vi "Initialize.vi"(8 "error in (no error)":errorcluster, 10 "Reply to":refnum<class "Result Reply Msg.lvclass">, 11 "Measure Controller in":refnum<class "Process Controller.lvclass">) -> (0 "error out":errorcluster, 3 "Measure Controller out":refnum<class "Process Controller.lvclass">)   [LabVIEW 2016, in "Process Controller.lvclass"]
uses:
  Process Controller.lvclass
  Measure Object Messages/Result Reply Msg/Result Reply Msg.lvclass
  Process Controller Messages/Init Response Msg/Init Response Msg.lvclass
  D:/github/Measure_core/Measure Object Messages/Result Reply Msg/Result Reply Msg.lvclass
  Results/Acquired Result/Acquired Result.lvclass
  Measure Object Messages/Initialize Msg/Initialize Msg.lvclass/Initialize Msg.ctl
  <vilib>/ActorFramework/Message Enqueuer/Message Enqueuer.lvclass/Message Enqueuer.ctl
  Process Controller.lvclass/Process Controller.ctl
  <vilib>/ActorFramework/Message Enqueuer/Enqueue.vi
  Measure Object Messages/Initialize Msg/Initialize Msg.lvclass
  D:/Program Files/National Instruments/LabVIEW 2016/vi.lib/ActorFramework/Message/Message.lvclass
  <vilib>/ActorFramework/Message Priority Queue/Priority Enqueue.vi
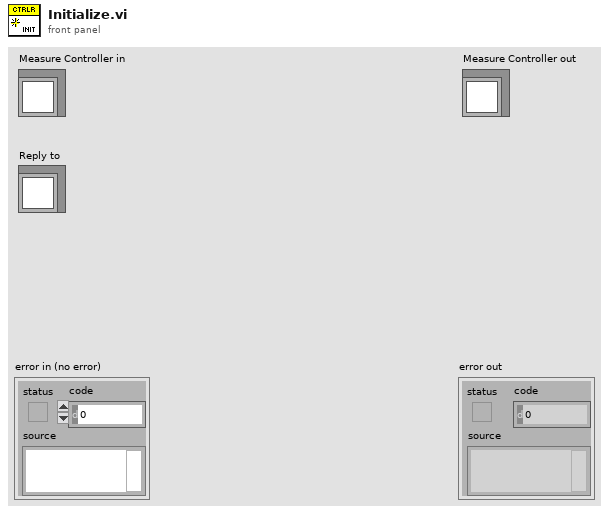
[diagram p1: front panel]
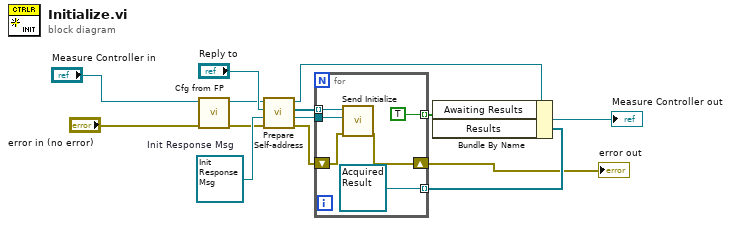
[diagram p0: block diagram]
diagram:
  w5 = refnum<class "Init Response Msg.lvclass"> refnum  # Init Response Msg
  n1 = call-dynamic "Cfg from FP.vi"("error in (no error)"="error in (no error)", "Measure Object in"="Measure Controller in") -> ("error out"=w3:errorcluster, "Measure Object out"=w1:refnum<class "Process Controller.lvclass">)  [unwired: 8 in]
  n2 = call-dynamic "Prepare Self-address.vi"("error in (no error)"=w3, "Reply to me"=w5, "Reply to"="Reply to", "Measure Controller in"=w1) -> ("error out"=w7:errorcluster, "Reply to me"=w9:refnum<class "Result Reply Msg.lvclass">, "Active measurements enqueuers"=w8:refnum<class "Message Enqueuer.lvclass">[], "Measure Controller out"=w6:refnum<class "Process Controller.lvclass">)  [unwired: 4 in]
  n3 = for {
    tunnel: w8 -> [w16] mode=indexing
    shift-right: [w20] -> w11
    shift-left: w7 -> [w15]
    tunnel: [TRUE] -> w14 mode=indexing
    tunnel: [refnum<class "Acquired Result.lvclass"> refnum ("Placeholder Result")] -> w13 mode=indexing
    tunnel: w9 -> [w17]
    n4 = call "Send Initialize.vi"("error in (no error)"=w15, "Reply to"=w17, "Message Enqueuer"=w16) -> ("error out"=w20:errorcluster)  [unwired: 7 in, 1 out]
  }
  "error out" <- w11
  n5 = Bundle By Name(cluster=w6, "Awaiting Results"=w14, "Results"=w13) -> (→"Measure Controller out":refnum<class "Process Controller.lvclass">)
